vi "Simple TCP - Client.vi"() -> ()   [LabVIEW 2019]
doc: "演示连接TCP服务器、读取发送的数据并在图表上显示数据的方法。VI设计为TCP连接断开时停止。"
panel:
  out "波形图表 3":i32(graph)
  in  "服务器关闭":string="服务器VI关闭了连接。"
  in  "停止":bool
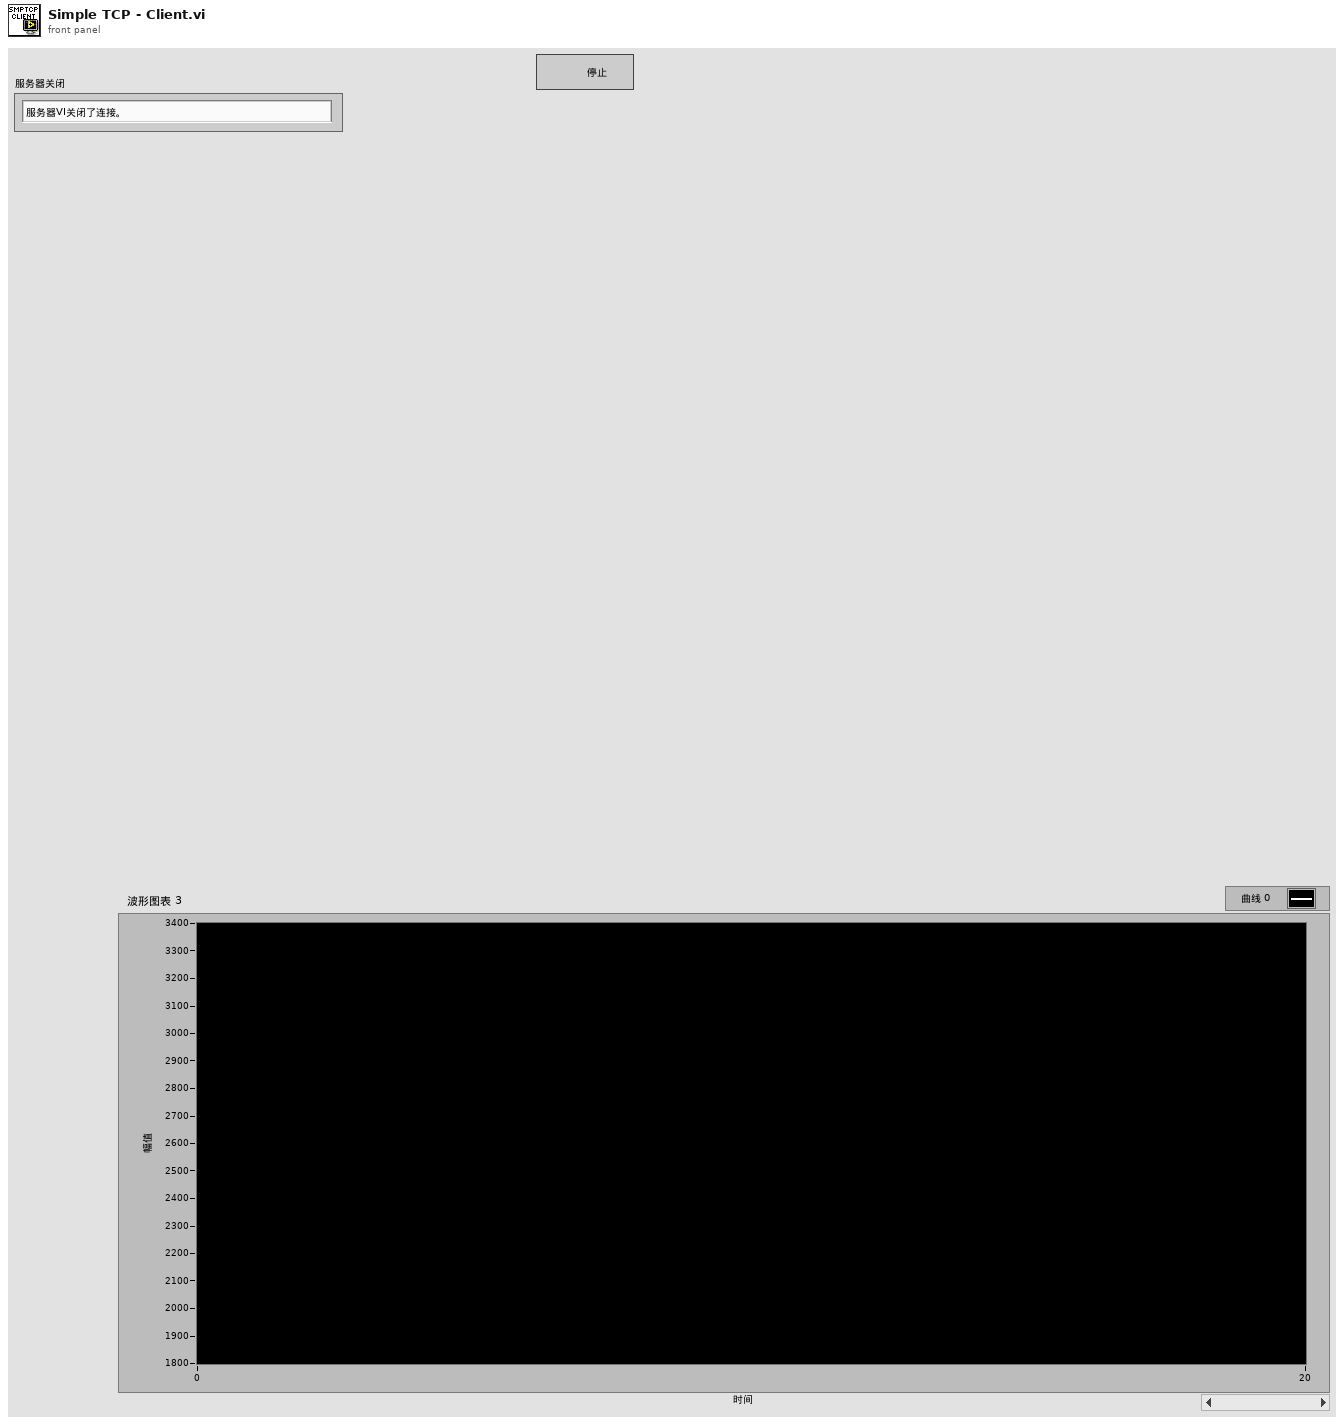
[diagram p1: front panel]
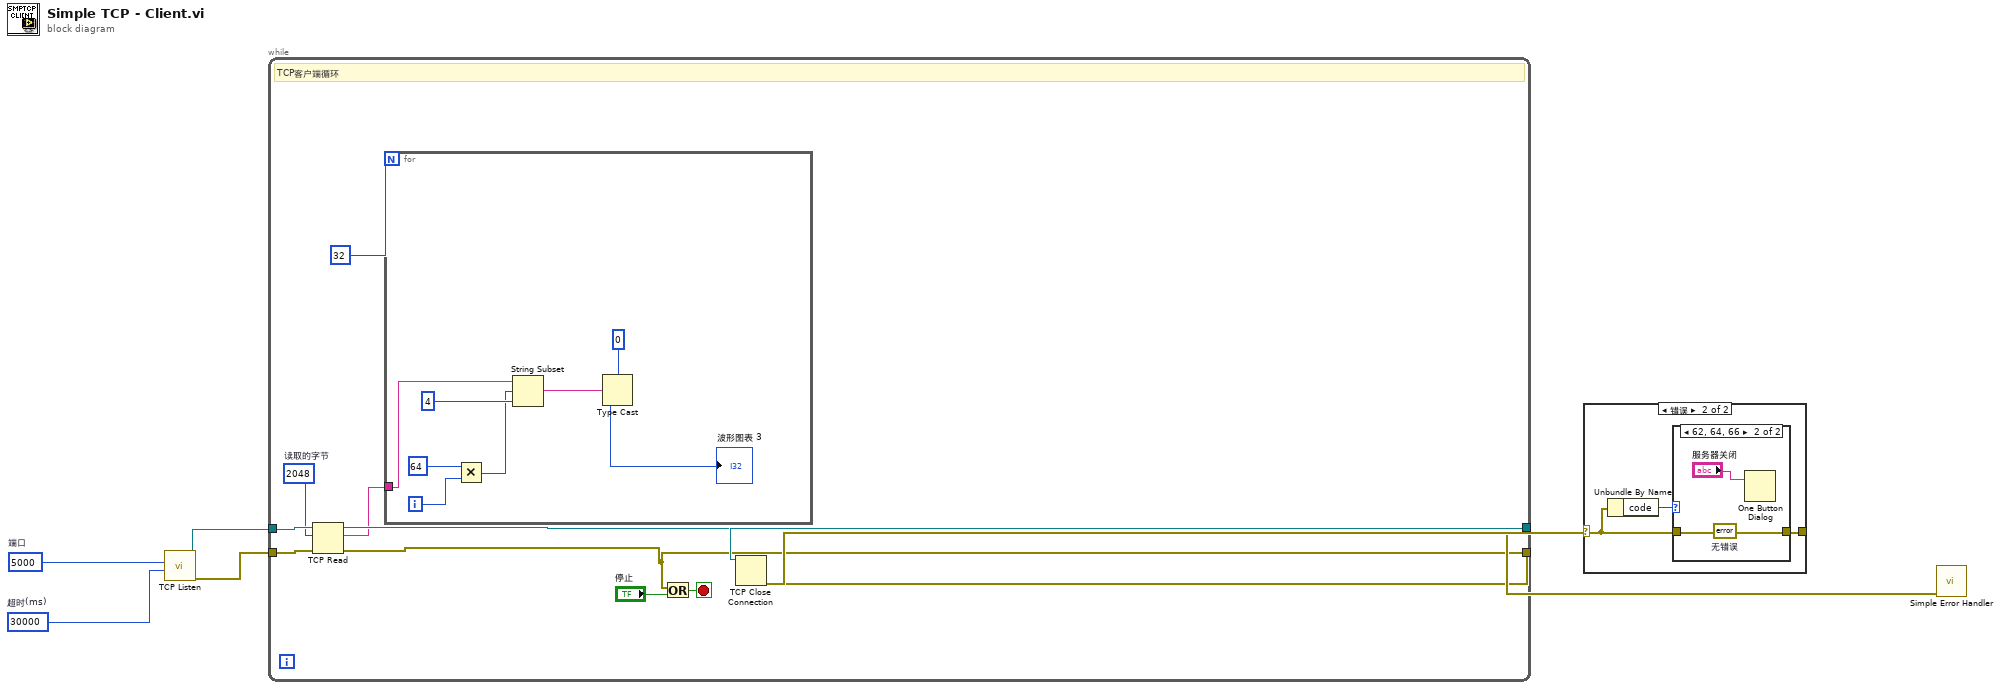
[diagram p0: block diagram]
diagram:
  w3 = u16 5000  # 端口
  w6 = 30000  # 超时(ms)
  n1 = call <vilib>:"TCP Listen.vi"("timeout ms (wait forever: -1)"=w6, "port"=w3) -> ("error out"=w4:errorcluster, "connection ID"=w5:refnum<k5>)  [unwired: 5 in, 3 out]
  n2 = while {
    tunnel: w4 -> [w16]
    tunnel: w5 -> [w17]
    tunnel: [w13] -> w2
    tunnel: [w12] -> w1
    stop <- w14 stop-if-true
    w11 = 2048  # 读取的字节
    # "TCP客户端循环"
    n3 = TCP Read(connection ID=w17, bytes to read=w11, error in (no error)=w16) -> (connection ID out=w13:refnum<k5>, data out=w10:string, error out=w12:errorcluster)  [unwired: 2 in]
    n4 = for {
      N: i8 32 -> [_]
      tunnel: w10 -> [w23]
      i -> [w22]
      n5 = Multiply(x=i8 64, y=w22) -> (x*y=w18:i32)
      n6 = String Subset(string=w23, offset (0)=w18, length (rest)=i8 4) -> (substring=w25:string)
      n7 = Type Cast(type=0, x=w25) -> (*(type *) &x=→"波形图表 3":i32)
    }
    n8 = Or(x=w12, y="停止") -> (x .or. y?=w14:bool)
  }
  n9 = TCP Close Connection(connection ID=w2, error in (no error)=w1) -> (error out=w8:errorcluster)  [unwired: 1 in, 1 out]
  n10 = case shown="错误" w8 {
    selector: w8 -> [w26 w28]
    tunnel: [w26 w27] -> w7
    frame No Error {
    }
    frame Error {
      n11 = Unbundle By Name(w28) -> ("code"=w29:i32)
      n12 = case shown="62, 64, 66" w29 {
        tunnel: w28 -> [w30 _]
        tunnel: [w30 w32] -> w27
        frame Default {
        }
        frame 62, 64, 66 {
          w32 = errorcluster {"status"=FALSE, "code"=0, "source"=""}  # 无错误
          n13 = One Button Dialog(message="服务器关闭") -> ()  [unwired: 1 in, 1 out]
        }
      }
    }
  }
  n14 = call <vilib>:"Simple Error Handler.vi"("error in (no error)"=w7) -> ()  [unwired: 4 in, 5 out]
